vi "guardadoarchivo.vi"(0 "nombre":string, 1 "lockin":dbl[][](array[numeric]), 2 "multimetro":bool, 3 "CCD":dbl[][](array[numeric]), 5 "titulo grupo":string, 7 "potenciometro":dbl[][](array[numeric]), 9 "Tipo de Medición":T1(ring), 11 "element":T2(ring), 12 "polarizador":dbl[][](array[numeric]), 13 "corriente":dbl[][](array[numeric]), 14 "multim.":dbl[][](array[numeric])) -> ()   [LabVIEW 2016]
doc: "En este subVI se realiza el guardado de la información de acuerdo con el dispositivo que se encuentre en penultimo lugar y si en ultimo lugar se encuentra la CCD. \n\nLas entradas son:\nLa cadena de nombre, en la que se especifica el nombre del archivo.\nLa cadena de nombre de los grupos que se van a realizar, en caso de que la cadena llegue vacía entoces no se forman ningún grupo."
uses:
  <vilib>/UPVI/lvhdf5/file.llb/LVH5F Operation.ctl
  <vilib>/Utility/miscctls.llb/LVRectTypeDef.ctl
  <vilib>/UPVI/lvhdf5/group.llb/H5G_obj_t.ctl
  <vilib>/UPVI/lvhdf5/dataset.llb/LVH5D Operation.ctl
  <vilib>/UPVI/lvhdf5/group.llb/OpenCreateGroup (String).vi
  <vilib>/UPVI/lvhdf5/utility.llb/Select HDF5 Dialog.vi
  <vilib>/UPVI/lvhdf5/utility.llb/Select HDF5 Dialog (Object Only).vi
  <vilib>/UPVI/lvhdf5/dataset.llb/Simple H5Dwrite (Variant).vi
  <vilib>/UPVI/lvhdf5/dataset.llb/Simple H5Dwrite.xnode
  <vilib>/UPVI/lvhdf5/library.llb/HDF5 Ref.ctl
  <vilib>/UPVI/lvhdf5/identifier.llb/Not an HDF5 Refnum Constant.vi
  <vilib>/Utility/error.llb/Error Cluster From Error Code.vi
  <vilib>/UPVI/lvhdf5/dataset.llb/OpenCreateReplace Dataset by Element Type.vi
  <vilib>/UPVI/lvhdf5/dataspace.llb/H5Sselect_hyperslab.vi
  <vilib>/UPVI/lvhdf5/dataset.llb/H5Dwrite (Variant).vi
  <vilib>/UPVI/lvhdf5/dataset.llb/H5Dget_space.vi
  <vilib>/UPVI/lvhdf5/attribute.llb/private/LVH5AwriteWDTAttrs.vi
  <vilib>/UPVI/lvhdf5/dataspace.llb/H5Sclose.vi
  <vilib>/UPVI/lvhdf5/dataset.llb/H5Dclose.vi
  <vilib>/UPVI/lvhdf5/utility.llb/Select HDF5 Dialog (File and Object).vi
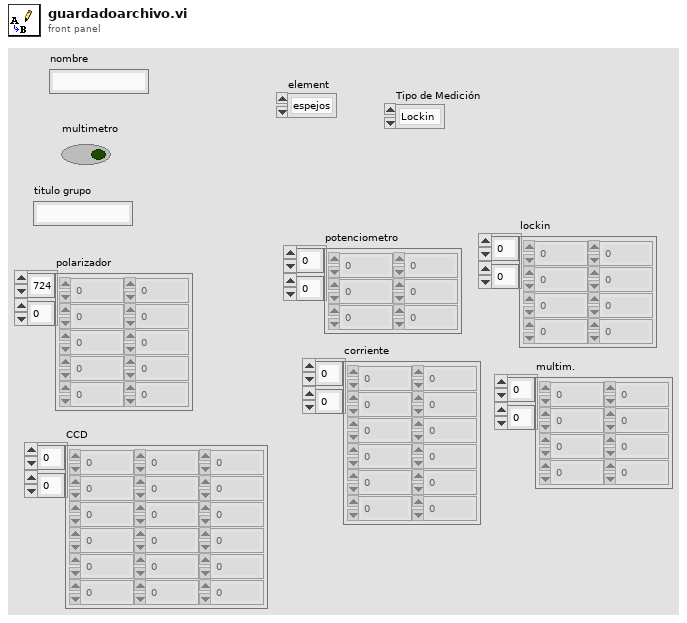
[diagram p1: front panel]
types:
  T1 = enum16{"Lockin", "Lockin-potenciometro", "Potenciometro"}
  T2 = enum16{"espejos", "polarizador", "voltaje", "potenciometro y lockin", "CCD"}
  T3 = typedef "LVH5F Operation.ctl" = enum16{"open", "open or create", "create or replace", "create or replace (with confirmation)", "create", "open (read only)"}
  T4 = typedef "HDF5 Ref.ctl" = refnum<k1>
  T5 = typedef "LVRectTypeDef.ctl" = cluster{"Left":i16, "Top":i16, "Right":i16, "Bottom":i16}
  T6 = cluster{"Behavior":enum32{"Invalid", "Default", "Floating", "Floating/Auto-Hide", "Modal"}, "Position":T5, "Center":bool, "Title":string}
  T7 = typedef "LVH5D Operation.ctl" = enum16{"open", "replace", "create", "open or create", "create or replace", "create or replace with confirmation"}
  T8 = typedef "H5G_obj_t.ctl" = i32
  T9 = cluster{"Object Types (any)":T8[], "Object Pattern":string}
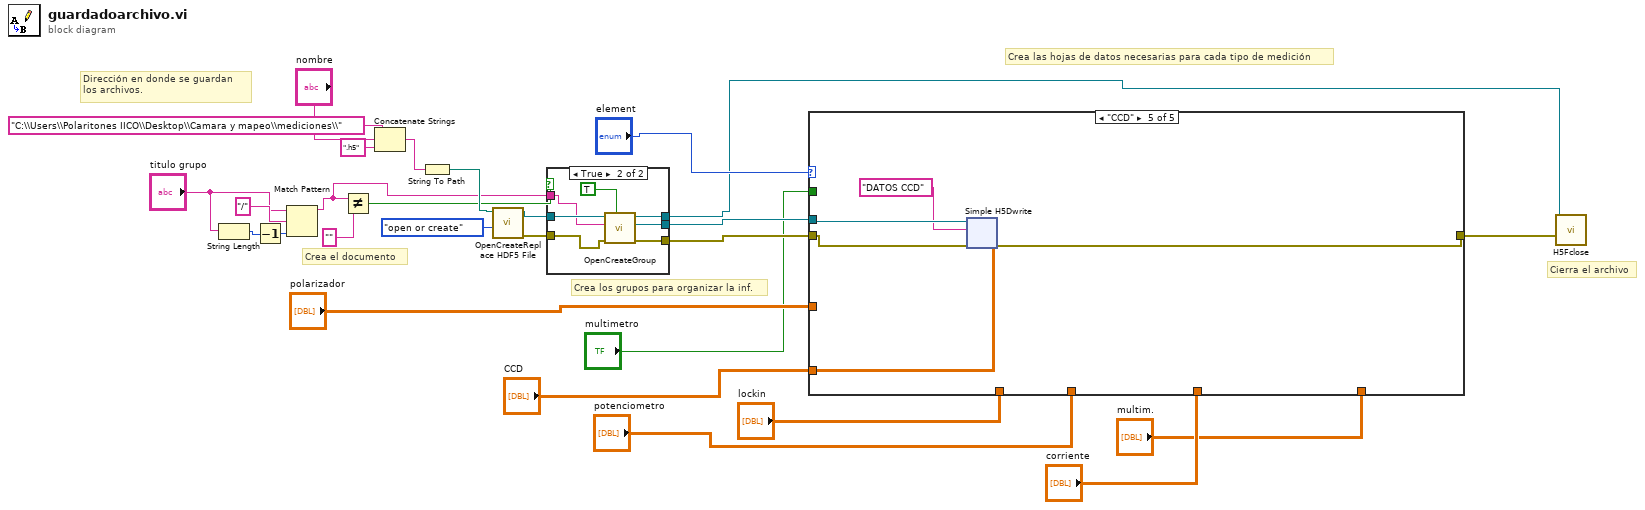
[diagram p0: block diagram]
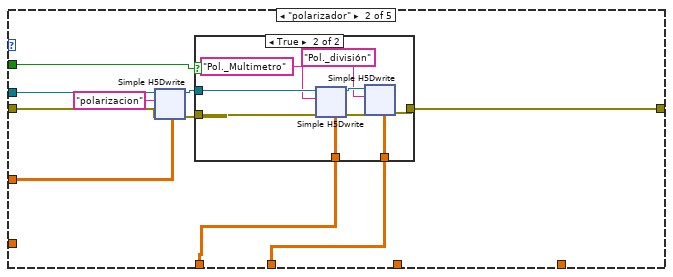
[diagram p4: hidden frame]
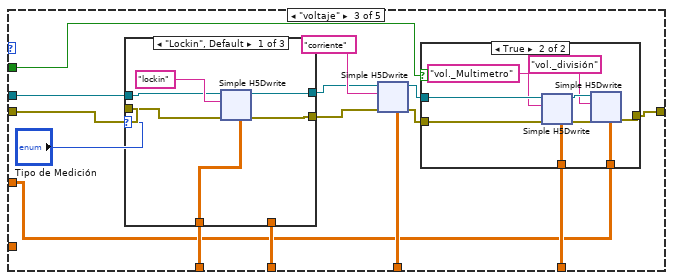
[diagram p6: hidden frame]
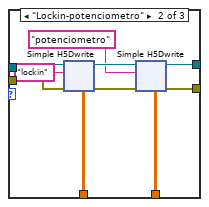
[diagram p8: hidden frame]
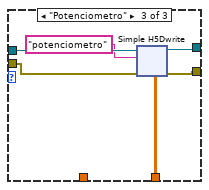
[diagram p9: hidden frame]
diagram:
  # "Dirección en donde se guardan \nlos archivos."
  # "Cierra el archivo"
  # "Crea las hojas de datos necesarias para cada tipo de medición"
  # "Crea los grupos para organizar la inf."
  # "Crea el documento"
  n1 = String Length(string="titulo grupo") -> (length=w8:i32)
  n2 = Decrement(x=w8) -> (x-1=w9:i32)
  n3 = Match Pattern(string="titulo grupo", regular expression="/", offset (0)=w9) -> (before substring=w4:string)  [unwired: 3 out]
  n4 = Not Equal?(x=w4, y="") -> (x != y?=w5:bool)
  n5 = Concatenate Strings("C:\\Users\\Polaritones IICO\\Desktop\\Camara y mapeo\\mediciones\\" ("string"), "nombre", ".h5" ("string")) -> (w21:string)
  n6 = String To Path(string=w21) -> (path=w20:path)
  n7 = call <vilib>:"OpenCreateReplace HDF5 File.vi"("function (open or create)"=LVH5F_Operation."open or create", "path"=w20) -> ("error out"=w25:errorcluster, "HDF5 Ref out"=w26:T4)  [unwired: 6 in]
  n8 = case shown="True" w5 {
    tunnel: w26 -> [w29 w36]
    tunnel: w25 -> [w28 w35]
    tunnel: [w28 w34] -> w19
    tunnel: [w29 w33] -> w17
    tunnel: [w29 w31] -> w15
    tunnel: w4 -> [_ w30]
    frame False {
    }
    frame True {
      n9 = call-poly <vilib>:"OpenCreateGroup.vi"("Create if not found (F)"=TRUE, "error in (no error)"=w35, "Group"=w30, "HDF5 Ref"=w36) -> ("error out"=w34:errorcluster, "HDF5 Group Ref"=w33:T4, "HDF5 Ref out"=w31:T4)  [unwired: 5 in]
    }
  }
  n10 = case shown="\"CCD\"" "element" {
    tunnel: w19 -> [w37 w47 w677 w2125 w2129]
    tunnel: "polarizador" -> [_ w46 w665 _ _]
    tunnel: w17 -> [_ w45 w678 _ w2128]
    tunnel: [w37 w41 w669 w2125 w2130] -> w14
    tunnel: "lockin" -> [_ w39 w676 _ _]
    tunnel: "potenciometro" -> [_ w38 w675 _ _]
    tunnel: "corriente" -> [_ _ w671 _ _]
    tunnel: "multimetro" -> [_ w40 w664 _ _]
    tunnel: "multim." -> [_ _ w666 _ _]
    tunnel: "CCD" -> [_ _ _ _ w2126]
    frame "espejos", Default {
    }
    frame "polarizador" {
      n11 = xnode "Simple H5Dwrite"("Dataset Path"="polarizacion", "error in (no error)"=w47, "HDF5 Path or Ref"=w45, "Data"=w46) -> ("HDF5 Ref out"=w42:T4, "error out"=w43:errorcluster)  [unwired: 4 in, 1 out]
      n12 = case shown="True" w40 {
        tunnel: w43 -> [w48 w57]
        tunnel: w42 -> [_ w56]
        tunnel: [w48 w52] -> w41
        tunnel: w39 -> [_ w50]
        tunnel: w38 -> [_ w49]
        frame False {
        }
        frame True {
          n13 = xnode "Simple H5Dwrite"("Dataset Path"="Pol._Multimetro", "error in (no error)"=w57, "HDF5 Path or Ref"=w56, "Data"=w50) -> ("HDF5 Ref out"=w53:T4, "error out"=w54:errorcluster)  [unwired: 4 in, 1 out]
          n14 = xnode "Simple H5Dwrite"("Dataset Path"="Pol._división", "error in (no error)"=w54, "HDF5 Path or Ref"=w53, "Data"=w49) -> ("error out"=w52:errorcluster)  [unwired: 4 in, 2 out]
        }
      }
    }
    frame "voltaje" {
      n15 = case shown="\"Lockin\", Default" "Tipo de Medición" {
        tunnel: w678 -> [w1299 w1511 w1919]
        tunnel: w677 -> [w1298 w1512 w1920]
        tunnel: w676 -> [w1295 w1509 _]
        tunnel: w675 -> [_ w1505 w1917]
        tunnel: [w1297 w1504 w1921] -> w674
        tunnel: [w1296 w1503 w1922] -> w672
        frame "Lockin", Default {
          n16 = xnode "Simple H5Dwrite"("Dataset Path"="lockin", "error in (no error)"=w1298, "HDF5 Path or Ref"=w1299, "Data"=w1295) -> ("HDF5 Ref out"=w1296:T4, "error out"=w1297:errorcluster)  [unwired: 4 in, 1 out]
        }
        frame "Lockin-potenciometro" {
          n17 = xnode "Simple H5Dwrite"("Dataset Path"="lockin", "error in (no error)"=w1512, "HDF5 Path or Ref"=w1511, "Data"=w1509) -> ("HDF5 Ref out"=w1508:T4, "error out"=w1507:errorcluster)  [unwired: 4 in, 1 out]
          n18 = xnode "Simple H5Dwrite"("Dataset Path"="potenciometro", "error in (no error)"=w1507, "HDF5 Path or Ref"=w1508, "Data"=w1505) -> ("HDF5 Ref out"=w1503:T4, "error out"=w1504:errorcluster)  [unwired: 4 in, 1 out]
        }
        frame "Potenciometro" {
          n19 = xnode "Simple H5Dwrite"("Dataset Path"="potenciometro", "error in (no error)"=w1920, "HDF5 Path or Ref"=w1919, "Data"=w1917) -> ("HDF5 Ref out"=w1922:T4, "error out"=w1921:errorcluster)  [unwired: 4 in, 1 out]
        }
      }
      n20 = xnode "Simple H5Dwrite"("Dataset Path"="corriente", "error in (no error)"=w674, "HDF5 Path or Ref"=w672, "Data"=w671) -> ("HDF5 Ref out"=w668:T4, "error out"=w667:errorcluster)  [unwired: 4 in, 1 out]
      n21 = case shown="True" w664 {
        tunnel: w667 -> [w679 w688]
        tunnel: w668 -> [_ w687]
        tunnel: [w679 w683] -> w669
        tunnel: w666 -> [_ w681]
        tunnel: w665 -> [_ w680]
        frame False {
        }
        frame True {
          n22 = xnode "Simple H5Dwrite"("Dataset Path"="vol._Multimetro", "error in (no error)"=w688, "HDF5 Path or Ref"=w687, "Data"=w681) -> ("HDF5 Ref out"=w684:T4, "error out"=w685:errorcluster)  [unwired: 4 in, 1 out]
          n23 = xnode "Simple H5Dwrite"("Dataset Path"="vol._división", "error in (no error)"=w685, "HDF5 Path or Ref"=w684, "Data"=w680) -> ("error out"=w683:errorcluster)  [unwired: 4 in, 2 out]
        }
      }
    }
    frame "potenciometro y lockin" {
    }
    frame "CCD" {
      n24 = xnode "Simple H5Dwrite"("Dataset Path"="DATOS CCD", "error in (no error)"=w2129, "HDF5 Path or Ref"=w2128, "Data"=w2126) -> ("error out"=w2130:errorcluster)  [unwired: 4 in, 2 out]
    }
  }
  n25 = call <vilib>:"H5Fclose.vi"("error in (no error)"=w14, "HDF5 Ref"=w15) -> ()  [unwired: 7 in, 1 out]
